vi "Get Models.vi"(8 "error in":errorcluster, 11 "AlicatCommBank in":refnum<class "AlicatCommBank.lvclass">=refnum) -> (0 "error out":errorcluster, 3 "AlicatCommBank out":refnum<class "AlicatCommBank.lvclass">)   [LabVIEW 2014, in "Alicat.lvlib" / "AlicatCommBank.lvclass"]
doc: "Request the model number of each of the devices in the Alicat Communication bank. Use this is you need to recast the devices."
uses:
  AlicatCommBank.lvclass
  Alicat.lvclass
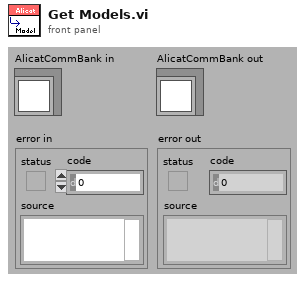
[diagram p1: front panel]
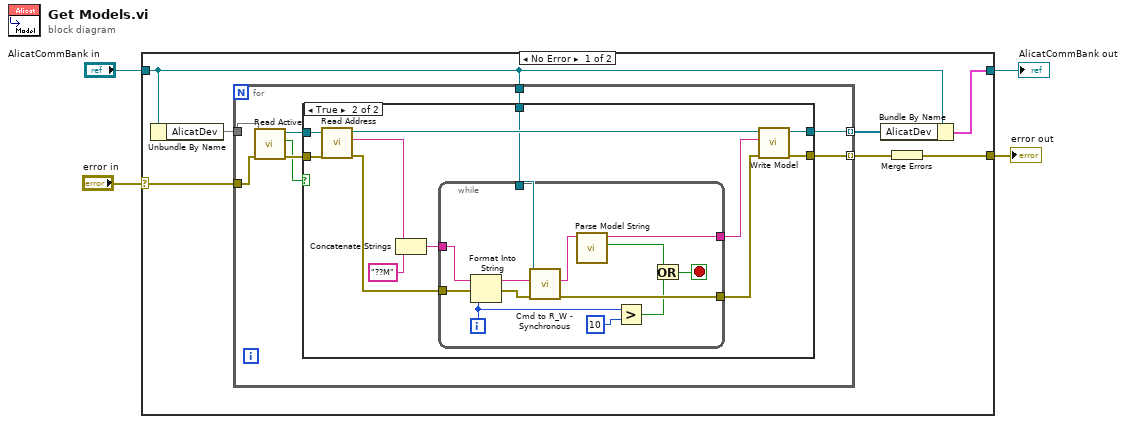
[diagram p0: block diagram]
diagram:
  n1 = case shown="No Error" "error in" {
    selector: "error in" -> [w10 w48]
    tunnel: [w9 w48] -> w3
    tunnel: [w7 w47] -> w1
    tunnel: "AlicatCommBank in" -> [w5 w47]
    frame No Error {
      n2 = Unbundle By Name(w5) -> ("AlicatDev"=w11)
      n3 = for {
        tunnel: w11 -> [w16]
        tunnel: w5 -> [w17]
        tunnel: w10 -> [w15]
        tunnel: [w19] -> w8 mode=indexing
        tunnel: [w18] -> w6 mode=indexing
        n4 = call "Read Active.vi"("error in"=w15, "Alicat in"=w16) -> ("error out"=w13:errorcluster, "Active?"=w12:bool, "Alicat out"=w14:refnum<class "Alicat.lvclass">)  [unwired: 7 in]
        n5 = case shown="True" w12 {
          tunnel: [w21 w32] -> w19
          tunnel: [w20 w31] -> w18
          tunnel: w17 -> [_ w29]
          tunnel: w14 -> [w21 w23]
          tunnel: w13 -> [w20 w22]
          frame False {
          }
          frame True {
            n6 = call "Read Address.vi"("error in"=w22, "Alicat in"=w23) -> ("error out"=w30:errorcluster, "Address"=w28:string, "Alicat out"=w33:refnum<class "Alicat.lvclass">)  [unwired: 7 in]
            n7 = Concatenate Strings(w28, "??M") -> (w26:string)
            n8 = while {
              tunnel: w26 -> [w46]
              tunnel: [w44] -> w25
              tunnel: [w43] -> w24
              tunnel: w30 -> [w42]
              tunnel: w29 -> [w41]
              i -> [w40]
              stop <- w36 stop-if-true
              n9 = Format Into String(initial string=w46, error in=w42, w40) -> (resulting string=w35:string, error out=w45:errorcluster)  [unwired: 1 in]
              n10 = call-dynamic "Cmd to R_W - Synchronous.vi"("error in"=w45, "write buffer"=w35, "Serial IO in"=w41) -> ("error out"=w43:errorcluster, "read buffer"=w34:string)  [unwired: 6 in, 1 out]
              n11 = call "Parse Model String.vi"("read buffer"=w34) -> ("Found?"=w38:bool, "token string"=w44:string)  [unwired: 9 in]
              n12 = Greater?(x=w40, y=10) -> (0:w37:bool)
              n13 = Or(x=w38, y=w37) -> (x .or. y?=w36:bool)
            }
            n14 = call "Write Model.vi"("error in"=w24, "Model"=w25, "Alicat in"=w33) -> ("error out"=w31:errorcluster, "Alicat out"=w32:refnum<class "Alicat.lvclass">)  [unwired: 7 in]
          }
        }
      }
      n15 = Bundle By Name(cluster=w5, "AlicatDev"=w8) -> (w7:cluster{})
      n16 = Merge Errors(w6) -> (w9:errorcluster)
    }
    frame Error {
    }
  }
  "error out" <- w3
  "AlicatCommBank out" <- w1
